vi "Get Topic Value.vi"(8 "error in (no error)":errorcluster, 9 "default value (empty variant)":variant, 10 "Topic":string, 11 "Communications in":refnum<class "Communications.lvclass">) -> (0 "error out":errorcluster, 1 "value":variant, 2 "found":bool, 3 "Communications out":refnum<class "Communications.lvclass">)   [LabVIEW 2019, in "Communications.lvclass"]
uses:
  Communications.lvclass
  Communications.lvclass/Communications.ctl
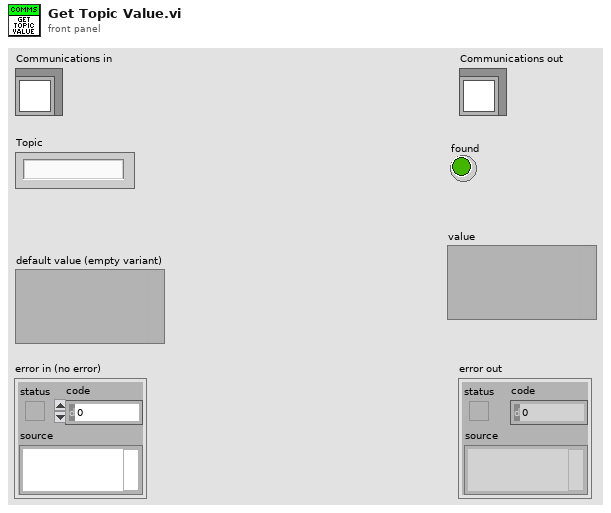
[diagram p1: front panel]
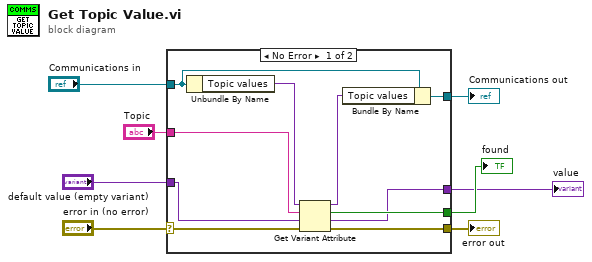
[diagram p0: block diagram]
diagram:
  n1 = case shown="No Error" "error in (no error)" {
    selector: "error in (no error)" -> [w16 w21]
    tunnel: [w14 w21] -> w7
    tunnel: [w13 w20] -> w5
    tunnel: "Communications in" -> [w18 w20]
    tunnel: "Topic" -> [w15 _]
    tunnel: [w11 _] -> w3
    tunnel: [w10 w19] -> w2
    tunnel: "default value (empty variant)" -> [w9 w19]
    frame No Error {
      n2 = Unbundle By Name(w18) -> ("Topic values"=w17:variant)
      n3 = Get Variant Attribute(Variant=w17, name=w15, default value (empty Variant)=w9, error in=w16) -> (duplicate Variant=w12:variant, found=w11:bool, value=w10:variant, error out=w14:errorcluster)
      n4 = Bundle By Name(cluster=w18, "Topic values"=w12) -> (w13:refnum<class "Communications.lvclass">)
    }
    frame Error {
    }
  }
  "error out" <- w7
  "Communications out" <- w5
  "value" <- w2
  "found" <- w3
